vi "Apply Highpass Filter_Frequency Domain.vi"(10 "cutoff frequency":dbl, 11 "spectrum":cluster{"f0":dbl, "df":dbl, "magnitude":sgl[]} {"magnitude" format="%.2f"; "df" format="%.2f"; "f0" format="%.2f"}) -> (3 "spectrum":cluster{"f0":dbl, "df":dbl, "magnitude":sgl[]})   [LabVIEW 2017, in "VibrationAnalysisFunctions.lvlib"]
uses:
  <vilib>/addons/InsightCM/Utilities/Analysis/Vibration/VibrationAnalysisFunctions.lvlib
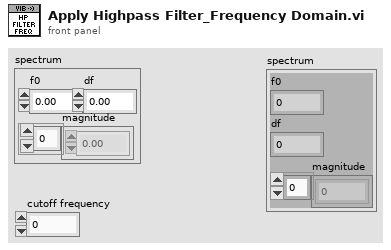
[diagram p1: front panel]
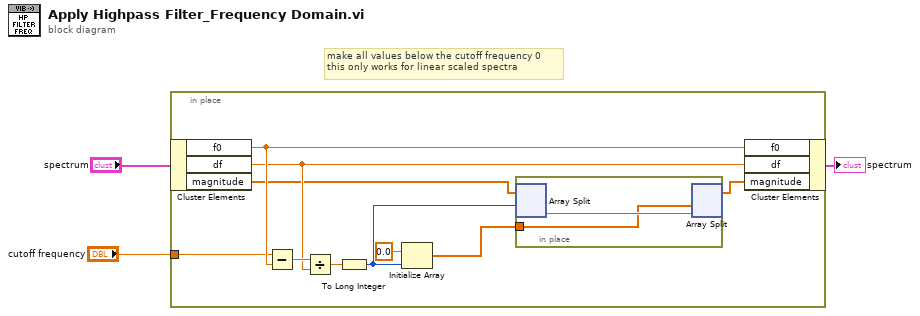
[diagram p0: block diagram]
diagram:
  # "make all values below the cutoff frequency 0\nthis only works for linear scaled spectra"
  n1 = in-place {
    in-place-border: "cutoff frequency" -> [w9]
    n2 = in-place-cluster #1("spectrum") -> ("f0"=w10:dbl, "df"=w8:dbl, "magnitude"=w6:sgl[])
    n3 = Subtract(x=w9, y=w10) -> (x-y=w13:dbl)
    n4 = Divide(x=w13, y=w8) -> (x/y=w12:dbl)
    n5 = To Long Integer(number=w12) -> (32bit integer=w7:i32)
    n6 = Initialize Array(sgl 0.0 ("element"), w7) -> (w5:sgl[])
    n7 = in-place {
      in-place-border: w5 -> [w14]
      n8 = in-place-split #2(w6, w7) -> (w15:sgl[])  [unwired: 1 out]
      n9 = in-place-split #2(w14, w15) -> (w4:sgl[])  [unwired: 1 out]
    }
    n10 = in-place-cluster #1("f0"=w10, "df"=w8, "magnitude"=w4) -> (→"spectrum":cluster{"f0":dbl, "df":dbl, "magnitude":sgl[]})
  }
